vi "Trav_cluster_Convert.vi"(4 "Traverse line in":T1 {"Row Duration (mins)" format="%#.1f"; "Row No" min=0; "Trace Gas Concentration (%)" min=0.0 format="%#.2f"; "Emission Rate (l/min)" format="%#.2f"; "Tunnel Speed" format="%#.2f"; "Start X" format="%#.2f"; "Start Y" format="%#.2f"; "Start Z" format="%#.2f"; "End X" format="%#.2f"; "End Y" format="%#.2f"; "End Z" format="%#.2f"; "Averaging time (min)" min=0.0 format="%#.2f"}, 5 "Channel Values In":string[](array[string]), 6 "Row Number":i32, 7 "Channel names":string[](array[string])) -> (0 "Traverse line Out":T1 {"Row Duration (mins)" format="%#.1f"; "Row No" min=0; "Trace Gas Concentration (%)" min=0.0 format="%#.2f"; "Emission Rate (l/min)" format="%#.2f"; "Tunnel Speed" format="%#.2f"; "Start X" format="%#.2f"; "Start Y" format="%#.2f"; "Start Z" format="%#.2f"; "End X" format="%#.2f"; "End Y" format="%#.2f"; "End Z" format="%#.2f"; "Averaging time (min)" min=0.0 format="%#.2f"})   [LabVIEW 2011]
uses:
  Traverse_cluster.ctl
  Spacing.ctl
  Controls/Multi_run_mode.ctl
  Globals/Trav_pos_global.vi
panel:
  # "X           Y            Z"
  # "Start"
  # "End"
  # "X           Y            Z"
  # "Start"
  # "End"
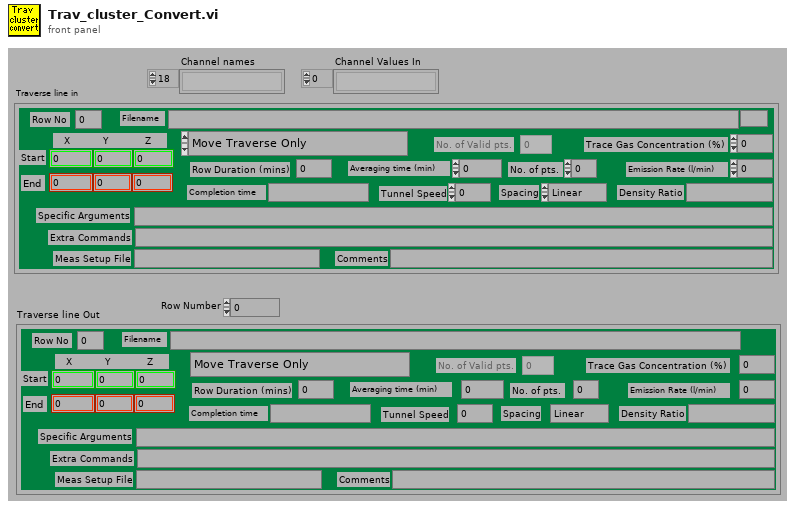
[diagram p1: front panel]
types:
  T1 = typedef "Traverse_cluster.ctl" = cluster{"Start X":dbl, "Start Y":dbl, "Start Z":dbl, "End X":dbl, "End Y":dbl, "End Z":dbl, "No. of pts.":i32, "Spacing":T2, "Filename":path, "Tunnel Speed":dbl, "Averaging time (min)":dbl, "Extra Commands":string, "Specific Arguments":string, "Emission Rate (l/min)":dbl, "Trace Gas Concentration (%)":dbl, "Density Ratio":string, "Comments":string, "Row No":i32, "Row Type Selector":T3, "Completion time":string, "Row Duration (mins)":dbl, "No. of Valid pts.":i32, "Meas Setup File":string}
  T2 = typedef "Spacing.ctl" = enum16{"Linear", "Log", "Gauss", "Specified", "N/A"}
  T3 = typedef "Multi_run_mode.ctl" = enum16{"Move Traverse Only", "Set Tunnel Speed Only", "Set Source Only", "Set Measurement Conditions", "Single Measurement", "Vertical Profile", "Lateral Profile", "Longitudinal Profile", "Explore Volume", "Multi-Axis Profile", "Auto Calibrate", "Meas Fast FID Bkgnd", "Check Beam Power", "Scanning Valve Measurement", "Run VI Named:", "Set ADAM Ch", "Wait (minutes)", "Send Message", "Synchronize With:", "Fall Back to this Row", "Turn Off Row Repeating", "Blank Row", "Traverse 3D Volume"}
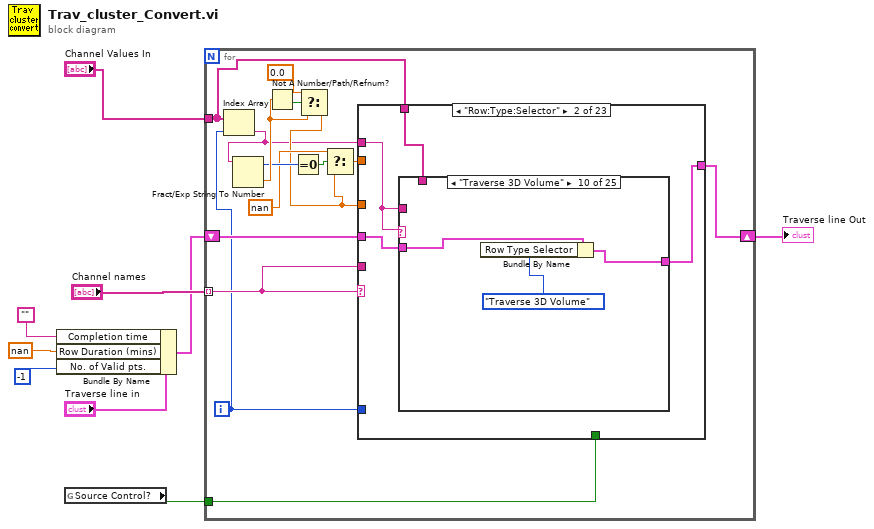
[diagram p0: block diagram]
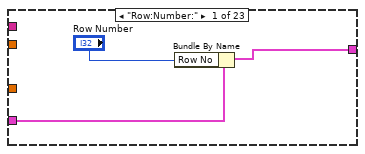
[diagram p2: hidden frame]
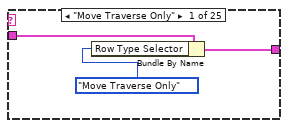
[diagram p3: hidden frame]
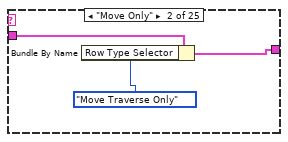
[diagram p4: hidden frame]
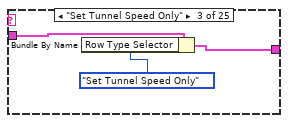
[diagram p5: hidden frame]
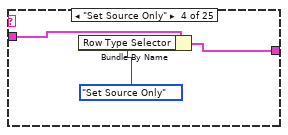
[diagram p6: hidden frame]
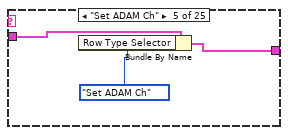
[diagram p7: hidden frame]
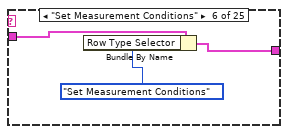
[diagram p8: hidden frame]
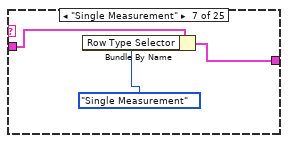
[diagram p9: hidden frame]
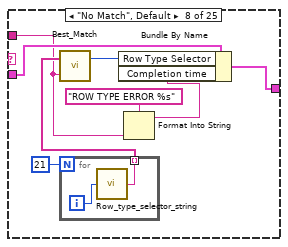
[diagram p10: hidden frame]
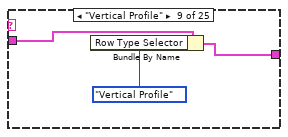
[diagram p11: hidden frame]
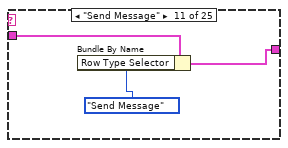
[diagram p12: hidden frame]
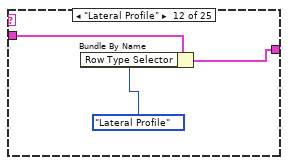
[diagram p13: hidden frame]
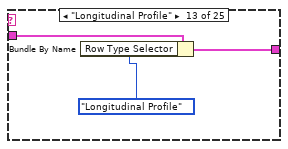
[diagram p14: hidden frame]
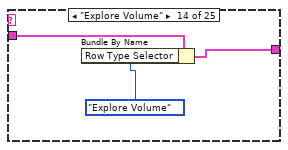
[diagram p15: hidden frame]
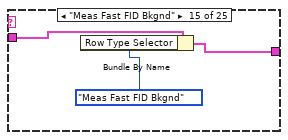
[diagram p16: hidden frame]
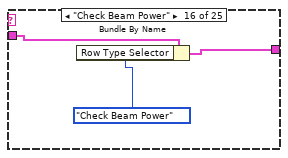
[diagram p17: hidden frame]
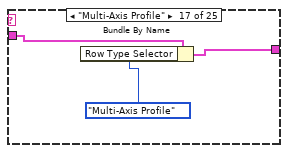
[diagram p18: hidden frame]
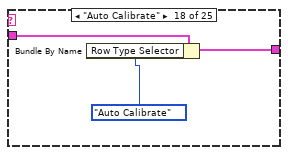
[diagram p19: hidden frame]
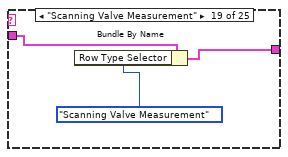
[diagram p20: hidden frame]
diagram:
  n1 = Bundle By Name(cluster="Traverse line in", "Completion time"="", "Row Duration (mins)"=nan ("Bundle Element"), "No. of Valid pts."=-1) -> (w4:T1)
  n2 = global read "Trav_pos_global.vi" "Source Control?"() -> (w9:bool)
  n3 = for {
    tunnel: "Channel names" -> [w14] mode=indexing
    shift-right: [w22] -> w3
    shift-left: w4 -> [w24]
    tunnel: w9 -> [w23]
    tunnel: "Channel Values In" -> [w10]
    i -> [w11]
    n4 = Index Array(array=w10, index=w11) -> (element=w12:string)
    n5 = Fract/Exp String To Number(string=w12) -> (offset past number=w18:i32, number=w20:dbl)  [unwired: 1 in, 2 out]
    n6 = Not A Number/Path/Refnum?(number/path/refnum=w20) -> (NaN/Path/Refnum?=w21:bool)
    n7 = Equal To 0?(x=w18) -> (x = 0?=w17:bool)
    n8 = Select(t=0.0, s=w21, f=w20) -> (s? t:f=w13:dbl)
    n9 = Select(t=nan ("f"), s=w17, f=w13) -> (s? t:f=w16:dbl)
    n10 = case shown="\"Row:Type:Selector\"" w14 {
      tunnel: w24 -> [w26 w30 w114 w118 w121 w125 w128 w130 w133 w135 w145 w151 w154 w159 w163 w166 w167 w170 w173 w179 w185 w186 w188]
      tunnel: w14 -> [_ _ _ _ _ _ _ _ _ _ _ _ _ _ _ _ _ _ _ _ _ _ w187]
      tunnel: w13 -> [_ _ w116 _ _ _ _ _ _ w138 _ w150 _ _ _ _ w169 w172 _ _ _ _ _]
      tunnel: [w27 w29 w115 w119 w122 w124 w127 w131 w134 w141 w144 w152 w157 w160 w162 w165 w168 w171 w175 w181 w185 w186 w188] -> w22
      tunnel: w12 -> [_ w31 _ _ _ _ _ _ _ _ w143 _ w156 w158 w161 w164 _ _ w174 w178 _ _ _]
      tunnel: w23 -> [_ _ _ _ _ _ _ _ _ _ _ _ _ _ _ _ _ _ _ _ _ _ _]
      tunnel: w11 -> [_ _ _ _ _ _ _ _ _ _ _ _ _ _ _ _ _ _ _ _ _ _ _]
      tunnel: w16 -> [_ _ _ w117 w120 w123 w126 w129 w132 _ _ _ _ _ _ _ _ _ _ _ _ _ _]
      tunnel: w10 -> [_ w28 _ _ _ _ _ _ _ _ _ _ _ _ _ _ _ _ _ w176 _ _ _]
      frame "Row:Number:" {
        n11 = Bundle By Name(cluster=w26, "Row No"="Row Number") -> (w27:T1)
      }
      frame "Row:Type:Selector" {
        n12 = case shown="\"Traverse 3D Volume\"" w31 {
          tunnel: w31 -> [_ _ _ _ _ _ _ w55 _ _ _ _ _ _ _ _ _ _ _ _ _ _ _ _ _]
          tunnel: w30 -> [w34 w36 w39 w42 w45 w48 w51 w57 w64 w67 w70 w74 w76 w80 w82 w85 w88 w92 w94 w97 w100 w103 w106 w109 w112]
          tunnel: [w33 w35 w38 w41 w44 w47 w50 w56 w65 w68 w69 w73 w75 w78 w81 w84 w87 w91 w93 w96 w99 w102 w105 w108 w113] -> w29
          tunnel: w28 -> [_ _ _ _ _ _ _ _ _ _ _ _ _ _ _ _ _ _ _ _ _ _ _ _ _]
          frame "Move Traverse Only" {
            n13 = Bundle By Name(cluster=w34, "Row Type Selector"=Multi_run_mode."Move Traverse Only" ("Mode")) -> (w33:T1)
          }
          frame "Move Only" {
            n14 = Bundle By Name(cluster=w36, "Row Type Selector"=Multi_run_mode."Move Traverse Only" ("Mode")) -> (w35:T1)
          }
          frame "Set Tunnel Speed Only" {
            n15 = Bundle By Name(cluster=w39, "Row Type Selector"=Multi_run_mode."Set Tunnel Speed Only" ("Mode")) -> (w38:T1)
          }
          frame "Set Source Only" {
            n16 = Bundle By Name(cluster=w42, "Row Type Selector"=Multi_run_mode."Set Source Only" ("Mode")) -> (w41:T1)
          }
          frame "Set ADAM Ch" {
            n17 = Bundle By Name(cluster=w45, "Row Type Selector"=Multi_run_mode."Set ADAM Ch" ("Mode")) -> (w44:T1)
          }
          frame "Set Measurement Conditions" {
            n18 = Bundle By Name(cluster=w48, "Row Type Selector"=Multi_run_mode."Set Measurement Conditions" ("Mode")) -> (w47:T1)
          }
          frame "Single Measurement" {
            n19 = Bundle By Name(cluster=w51, "Row Type Selector"=Multi_run_mode."Single Measurement" ("Mode")) -> (w50:T1)
          }
          frame "No Match", Default {
            n20 = for {
              N: 21 -> [_]
              tunnel: [w61] -> w59 mode=indexing
              i -> [w62]
              n21 = call "Row_type_selector_string.vi"("Mode"=w62) -> ("Output string"=w61:string)
            }
            n22 = call "Best_Match.vi"("Input String"=w55, "String Options"=w59) -> ("index of element"=w58:i32)  [unwired: 1 out]
            n23 = Format Into String(format string="ROW TYPE ERROR %s", w55) -> (resulting string=w53:string)  [unwired: 2 in, 1 out]
            n24 = Bundle By Name(cluster=w57, "Row Type Selector"=w58, "Completion time"=w53) -> (w56:T1)
          }
          frame "Vertical Profile" {
            n25 = Bundle By Name(cluster=w64, "Row Type Selector"=Multi_run_mode."Vertical Profile" ("Mode")) -> (w65:T1)
          }
          frame "Traverse 3D Volume" {
            n26 = Bundle By Name(cluster=w67, "Row Type Selector"=Multi_run_mode."Traverse 3D Volume" ("Mode")) -> (w68:T1)
          }
          frame "Send Message" {
            n27 = Bundle By Name(cluster=w70, "Row Type Selector"=Multi_run_mode."Send Message" ("Mode")) -> (w69:T1)
          }
          frame "Lateral Profile" {
            n28 = Bundle By Name(cluster=w74, "Row Type Selector"=Multi_run_mode."Lateral Profile" ("Mode")) -> (w73:T1)
          }
          frame "Longitudinal Profile" {
            n29 = Bundle By Name(cluster=w76, "Row Type Selector"=Multi_run_mode."Longitudinal Profile" ("Mode")) -> (w75:T1)
          }
          frame "Explore Volume" {
            n30 = Bundle By Name(cluster=w80, "Row Type Selector"=Multi_run_mode."Explore Volume" ("Mode")) -> (w78:T1)
          }
          frame "Meas Fast FID Bkgnd" {
            n31 = Bundle By Name(cluster=w82, "Row Type Selector"=Multi_run_mode."Meas Fast FID Bkgnd" ("Mode")) -> (w81:T1)
          }
          frame "Check Beam Power" {
            n32 = Bundle By Name(cluster=w85, "Row Type Selector"=Multi_run_mode."Check Beam Power" ("Mode")) -> (w84:T1)
          }
          frame "Multi-Axis Profile" {
            n33 = Bundle By Name(cluster=w88, "Row Type Selector"=Multi_run_mode."Multi-Axis Profile" ("Mode")) -> (w87:T1)
          }
          frame "Auto Calibrate" {
            n34 = Bundle By Name(cluster=w92, "Row Type Selector"=Multi_run_mode."Auto Calibrate" ("Mode")) -> (w91:T1)
          }
          frame "Scanning Valve Measurement" {
            n35 = Bundle By Name(cluster=w94, "Row Type Selector"=Multi_run_mode."Scanning Valve Measurement" ("Mode")) -> (w93:T1)
          }
          frame "Wait (minutes)" {
            n36 = Bundle By Name(cluster=w97, "Row Type Selector"=Multi_run_mode."Wait (minutes)" ("Mode")) -> (w96:T1)
          }
          frame "Run VI Named:" {
            n37 = Bundle By Name(cluster=w100, "Row Type Selector"=Multi_run_mode."Run VI Named:" ("Mode")) -> (w99:T1)
          }
          frame "Synchronize With:" {
            n38 = Bundle By Name(cluster=w103, "Row Type Selector"=Multi_run_mode."Synchronize With:" ("Mode")) -> (w102:T1)
          }
          frame "Fall Back to this Row" {
            n39 = Bundle By Name(cluster=w106, "Row Type Selector"=Multi_run_mode."Fall Back to this Row" ("Mode")) -> (w105:T1)
          }
          frame "Turn Off Row Repeating" {
            n40 = Bundle By Name(cluster=w109, "Row Type Selector"=Multi_run_mode."Turn Off Row Repeating" ("Mode")) -> (w108:T1)
          }
          frame "" {
            n41 = Bundle By Name(cluster=w112, "Row Type Selector"=Multi_run_mode."Blank Row" ("Mode")) -> (w113:T1)
          }
        }
      }
      frame "Tunnel:Speed:(m/s)" {
        n42 = Bundle By Name(cluster=w114, "Tunnel Speed"=w116) -> (w115:T1)
      }
      frame "Start at:X:(mm)" {
        n43 = Bundle By Name(cluster=w118, "Start X"=w117) -> (w119:T1)
      }
      frame "Start at:Y:(mm)" {
        n44 = Bundle By Name(cluster=w121, "Start Y"=w120) -> (w122:T1)
      }
      frame "Start at:Z:(mm)" {
        n45 = Bundle By Name(cluster=w125, "Start Z"=w123) -> (w124:T1)
      }
      frame "End at:X:(mm)" {
        n46 = Bundle By Name(cluster=w128, "End X"=w126) -> (w127:T1)
      }
      frame "End at:Y:(mm)" {
        n47 = Bundle By Name(cluster=w130, "End Y"=w129) -> (w131:T1)
      }
      frame "End at:Z:(mm)" {
        n48 = Bundle By Name(cluster=w133, "End Z"=w132) -> (w134:T1)
      }
      frame "Number:Of:Points" {
        n49 = Not A Number/Path/Refnum?(number/path/refnum=w138) -> (NaN/Path/Refnum?=w140:bool)
        n50 = To Long Integer(number=w138) -> (32bit integer=w139:i32)
        n51 = Select(t=0, s=w140, f=w139) -> (s? t:f=w136:i32)
        n52 = Bundle By Name(cluster=w135, "No. of pts."=w136) -> (w141:T1)
      }
      frame "Point:Spacing:Method" {
        n53 = case shown="\"Linear\", Default" w143 {
          tunnel: [Spacing."Linear" ("Spacing") Spacing."Log" ("Spacing") Spacing."Gauss" ("Spacing") Spacing."Specified" ("Spacing")] -> w142
          frame "Linear", Default {
          }
          frame "Log" {
          }
          frame "Gauss" {
          }
          frame "Specified" {
          }
        }
        n54 = Bundle By Name(cluster=w145, "Spacing"=w142) -> (w144:T1)
      }
      frame "Averaging:Time:(mins)" {
        n55 = Bundle By Name(cluster=w151, "Averaging time (min)"=w150) -> (w152:T1)
      }
      frame "Filename:HD:Users" {
        n56 = call "Text_without_format.vi"("Input string"=w156) -> ("Output string"=w155:string)
        n57 = String To Path(string=w155) -> (path=w153:path)
        n58 = Bundle By Name(cluster=w154, "Filename"=w153) -> (w157:T1)
      }
      frame "Specific:Arguments:String" {
        n59 = Bundle By Name(cluster=w159, "Specific Arguments"=w158) -> (w160:T1)
      }
      frame "Measurement:Setup:File" {
        n60 = Bundle By Name(cluster=w163, "Meas Setup File"=w161) -> (w162:T1)
      }
      frame "Extra:Commands:String" {
        n61 = Bundle By Name(cluster=w166, "Extra Commands"=w164) -> (w165:T1)
      }
      frame "Emission:Rate:(l/min)" {
        n62 = Bundle By Name(cluster=w167, "Emission Rate (l/min)"=w169) -> (w168:T1)
      }
      frame "Trace Gas:Concentration:(%)" {
        n63 = Bundle By Name(cluster=w170, "Trace Gas Concentration (%)"=w172) -> (w171:T1)
      }
      frame "Density:Ratio:" {
        n64 = Bundle By Name(cluster=w173, "Density Ratio"=w174) -> (w175:T1)
      }
      frame "Comments::" {
        n65 = Unbundle By Name(w179) -> ("Row Type Selector"=w180:T3)
        n66 = case shown="\"Blank Row\"" w180 {
          tunnel: [w182 w183] -> w177
          tunnel: w178 -> [w182 _]
          tunnel: w176 -> [_ w184]
          frame "Set ADAM Ch", Default {
          }
          frame "Blank Row" {
            n67 = Concatenate Strings(w184) -> (w183:string)
          }
        }
        n68 = Bundle By Name(cluster=w179, "Comments"=w177) -> (w181:T1)
      }
      frame "Row:Completion:Time" {
      }
      frame "Time:Taken in:Row (mins)" {
      }
      frame "No match", Default {
        n69 = call "Was_string_matched.vi"("Variable name"=w187) -> ()  [unwired: 2 in]
      }
    }
  }
  "Traverse line Out" <- w3
